vi "2021 Advent puzzle 06.vi"() -> ()   [LabVIEW 2021]
panel:
  out "Previous sum":u64=1593993084459
  out "overflow":bool
  in  "days":i32=256
  out "sum":u64=1754000560399
  out "Count":i32=255
  out "Lanterfishes":u64[](array[numeric])=[146420535621, 181966821442, 187095553356, 200982042686, 238871757043, 225243895868, 293366118418, 120046360025, 160007475940]
  in  "Test":bool
  # "after 18 days, there are a total of 26 fish. After 80 days, there would be a total of 5934"
  # "After 256 days in the example above, there would be a total of 26984457539 lanternfish!"
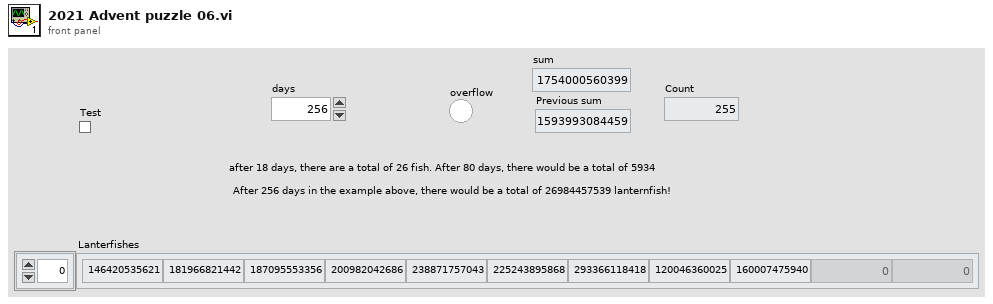
[diagram p1: front panel]
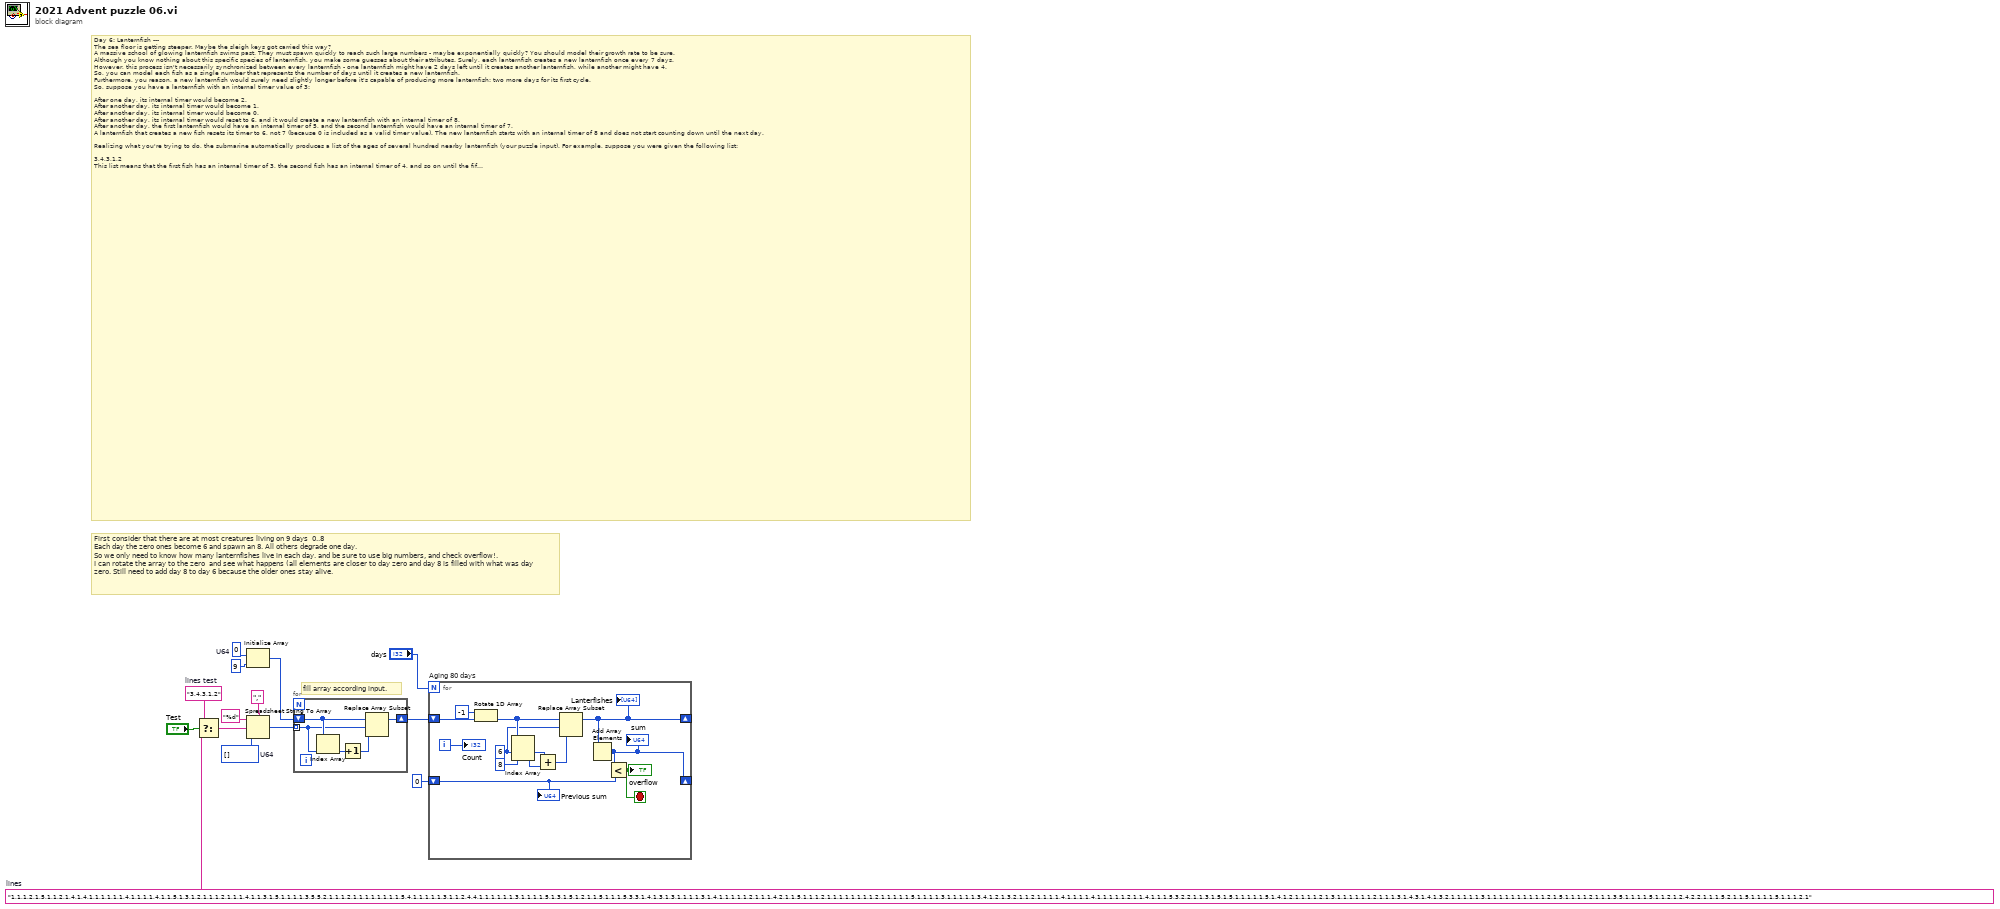
[diagram p0: block diagram]
diagram:
  w6 = u64 0  # U64
  w9 = u64[] []  # U64
  w14 = "3,4,3,1,2"  # lines test
  w12 = "1,1,1,2,1,5,1,1,2,1,4,1,4,1,1,1,1,1,1,4,1,1,1,1,4,1,1,5,1,3,1,2,1,1,1,2,1,1,1,4,1,1,3,1,5,1,1,1,1,3,5,5,2,1,1,1,2,1,1,1,1,1,1,1,1,5,4,1,1,1,1,1,3,1,1,2,4,4,1,1,1,1,1,1,3,1,1,1,1,5,1,3,1,5,1,2,1,1,5,1,1,1,5,3,3,1,4,1,3,1,3,1,1,1,1,3,1,4,1,1,1,1,1,2,1,1,1,4,2,1,1,5,1,1,1,2,1,1,1,1,1,1,1,1,2,1,1,1,1,1,5,1,1,1,1,3,1,1,1,1,1,3,4,1,2,1,3,2,1,1,2,1,1,1,1,4,1,1,1,1,4,1,1,1,1,1,2,1,1,4,1,1,1,5,3,2,2,1,1,3,1,5,1,5,1,1,1,1,1,5,1,4,1,2,1,1,1,1,2,1,3,1,1,1,1,1,1,2,1,1,1,3,1,4,3,1,4,1,3,2,1,1,1,1,1,3,1,1,1,1,1,1,1,1,1,1,2,1,5,1,1,1,1,2,1,1,1,3,5,1,1,1,1,5,1,1,2,1,2,4,2,2,1,1,1,5,2,1,1,5,1,1,1,1,5,1,1,1,2,1"  # lines
  # "fill array according input."
  # "First consider that there are at most creatures living on 9 days  0..8\nEach day the zero ones become 6 and spawn an 8. All others degrade one day.\nSo we only need to know how many lanternfishes live in each day. and be sure to use big numbers, and check overflow!.\nI can rotate the array to the zero  and see what happens (all elements are closer to day zero and day 8 is filled with what was day zero. Still need to add day 8 to day 6 because the older ones stay alive."
  # "Day 6: Lanternfish ---\nThe sea floor is getting steeper. Maybe the sleigh keys got carried this way?\nA massive school of glowing lanternfish swims past. They must spawn quickly to reach such large numbers - maybe exponentially quickly? You should model their growth rate to be sure.\nAlthough you know nothing about this specific species of lanternfish, you make some guesses about their attributes. Surely, each lanternfish creates a new lanternfish once every 7 days.\nHowever, this process isn't necessarily synchronized between every lanternfish - one lanternfish might have 2 days left until it creates another lanternfish, while another might have 4. \nSo, you can model each fish as a single number that represents the number of days until it creates a new lanternfish.\nFurthermore, you reason, a new lanternfish would surely need slightly longer before it's capable of producing more lanternfish: two more days for its first cycle.\nSo, suppose you have a lanternfish with an internal timer value of 3:\n\nAfter one day, its internal timer would become 2.\nAfter another day, its internal timer would become 1.\nAfter another day, its internal timer would become 0.\nAfter another day, its internal timer would reset to 6, and it would create a new lanternfish with an internal timer of 8.\nAfter another day, the first lanternfish would have an internal timer of 5, and the second lanternfish would have an internal timer of 7.\nA lanternfish that creates a new fish resets its timer to 6, not 7 (because 0 is included as a valid timer value). The new lanternfish starts with an internal timer of 8 and does not start counting down until the next day.\n\nRealizing what you're trying to do, the submarine automatically produces a list of the ages of several hundred nearby lanternfish (your puzzle input). For example, suppose you were given the following list:\n\n3,4,3,1,2\nThis list means that the first fish has an internal timer of 3, the second fish has an internal timer of 4, and so on until the fifth fish, which has an internal timer of 2. Simulating these fish over several days would proceed as follows:\n Initial state: 3,4,3,1,2\nAfter  1 day:  2,3,2,0,1\nAfter  2 days: 1,2,1,6,0,8\nAfter  3 days: 0,1,0,5,6,7,8\nAfter  4 days: 6,0,6,4,5,6,7,8,8\nAfter  5 days: 5,6,5,3,4,5,6,7,7,8\nAfter  6 days: 4,5,4,2,3,4,5,6,6,7\nAfter  7 days: 3,4,3,1,2,3,4,5,5,6\nAfter  8 days: 2,3,2,0,1,2,3,4,4,5\nAfter  9 days: 1,2,1,6,0,1,2,3,3,4,8\nAfter 10 days: 0,1,0,5,6,0,1,2,2,3,7,8\nAfter 11 days: 6,0,6,4,5,6,0,1,1,2,6,7,8,8,8\nAfter 12 days: 5,6,5,3,4,5,6,0,0,1,5,6,7,7,7,8,8\nAfter 13 days: 4,5,4,2,3,4,5,6,6,0,4,5,6,6,6,7,7,8,8\nAfter 14 days: 3,4,3,1,2,3,4,5,5,6,3,4,5,5,5,6,6,7,7,8\nAfter 15 days: 2,3,2,0,1,2,3,4,4,5,2,3,4,4,4,5,5,6,6,7\nAfter 16 days: 1,2,1,6,0,1,2,3,3,4,1,2,3,3,3,4,4,5,5,6,8\nAfter 17 days: 0,1,0,5,6,0,1,2,2,3,0,1,2,2,2,3,3,4,4,5,7,8\nAfter 18 days: 6,0,6,4,5,6,0,1,1,2,6,0,1,1,1,2,2,3,3,4,6,7,8,8,8,8\nEach day, a 0 becomes a 6 and adds a new 8 to the end of the list, while each other number decreases by 1 if it was present at the start of the day.\n\nIn this example, after 18 days, there are a total of 26 fish. After 80 days, there would be a total of 5934.\n\nFind a way to simulate lanternfish. How many lanternfish would there be after 80 days?"
  n1 = Select(t=w14, s="Test", f=w12) -> (s? t:f=w8:string)
  n2 = Initialize Array(w6, 9 ("dimension size")) -> (w4:u64[])
  n3 = Spreadsheet String To Array(delimiter (Tab)=",", format string="%d", spreadsheet string=w8, array type (2D Dbl)=w9) -> (array=w5:u64[])
  n4 = for {
    tunnel: w5 -> [w17] mode=indexing
    shift-right: [w19] -> w3
    shift-left: w4 -> [w18]
    n5 = Index Array(array=w18, index=w17) -> (element=w16:u64)
    n6 = Increment(x=w16) -> (x+1=w15:u64)
    n7 = Replace Array Subset(array=w18, new element=w15, index=w17) -> (w19:u64[])
  }
  n8 = for "Aging 80 days" {
    N: "days" -> [_]
    shift-right: [w23] -> _
    shift-left: w3 -> [w31]
    shift-right: [w22] -> _
    shift-left: u64 0 ("U64") -> [w21]
    i -> [w32]
    stop <- w20 stop-if-true
    w24 = 6 ("index")
    n9 = Rotate 1D Array(1:w31, 2:-1 ("n")) -> (0:w29:u64[])
    n10 = Index Array(array=w29, index #1=w24, index #2=8 ("index")) -> (element #1=w27:u64, element #2=w26:u64)
    n11 = Add(x=w27, y=w26) -> (x+y=w25:u64)
    n12 = Replace Array Subset(array=w29, new element=w25, index=w24) -> (w23:u64[])
    "Lanterfishes" <- w23
    n13 = Add Array Elements(numeric array=w23) -> (sum=w22:u64)
    "sum" <- w22
    n14 = Less?(x=w22, y=w21) -> (x < y?=w20:bool)
    "overflow" <- w20
    "Count" <- w32
    "Previous sum" <- w21
  }
